vi "NewTemplate.CreateBroadcasts.vi"(8 "error in (no error)":errorcluster) -> (0 "error out":errorcluster, 3 "Broadcasts":T1)   [LabVIEW 2024, in "ModuleManager.lvclass"]
uses:
  ModuleManager.lvclass
  Broadcast Events--cluster.ctl
  Stopped.ctl
  ModuleManager.lvclass/ModuleManager.ctl
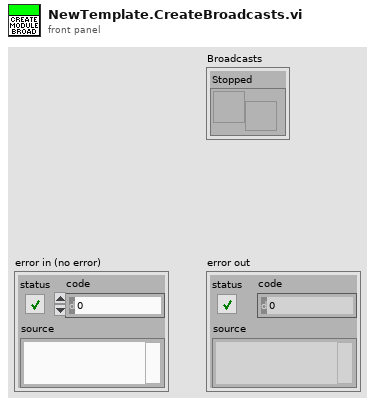
[diagram p1: front panel]
types:
  T1 = typedef "ModuleManager.lvclass/Broadcast Events--cluster.ctl" = cluster{"Stopped":refnum<user-event>}
  T2 = typedef "ModuleManager.lvclass/Stopped.ctl" = bool
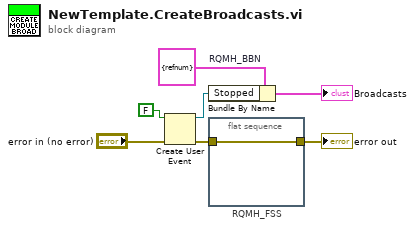
[diagram p0: block diagram]
diagram:
  n1 = Create User Event(user event datatype=T2 FALSE ("Stopped"), error in="error in (no error)") -> (user event=w6:refnum<user-event>, error out=w1:errorcluster)
  n2 = Bundle By Name "RQMH_BBN"(cluster=T1 {"Stopped"=refnum} ("Broadcasts"), "Stopped"=w6) -> (→"Broadcasts":T1)
  n3 = flat-sequence "RQMH_FSS" {
    tunnel: w1 -> [w8]
    tunnel: [w8] -> w2
    frame #0 {
    }
  }
  "error out" <- w2
